vi "Snoothing.vi"(0 "Output 2":refnum<vi>, 2 "Value":i32, 3 "Delay (ms)":u32) -> (1 "Output":i32)   [LabVIEW 2015]
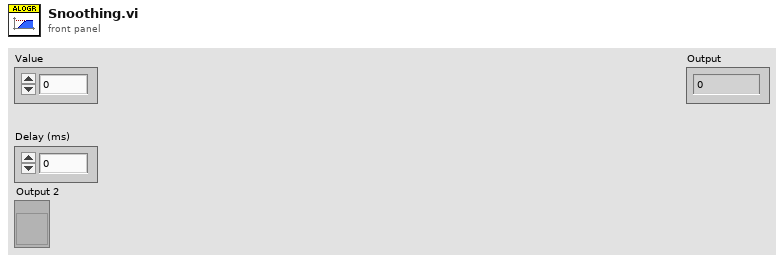
[diagram p1: front panel]
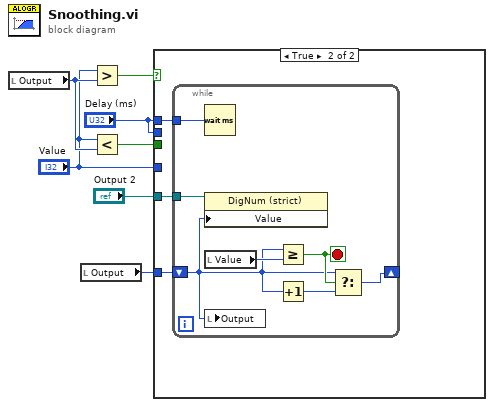
[diagram p0: block diagram]
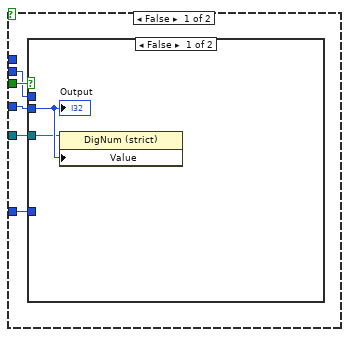
[diagram p2: hidden frame]
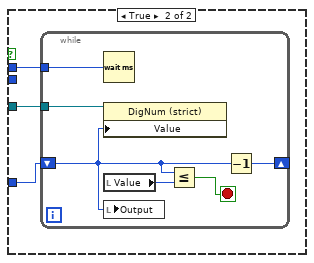
[diagram p3: hidden frame]
diagram:
  n1 = local read "Output"() -> (w6:i32)
  n2 = local read "Output"() -> (w4:i32)
  n3 = Greater?(x="Value", y=w6) -> (0:w7:bool)
  n4 = Less?(x="Value", y=w6) -> (x < y?=w5:bool)
  n5 = case shown="True" w7 {
    tunnel: w5 -> [w12 _]
    tunnel: w4 -> [w11 w26]
    tunnel: "Value" -> [w10 _]
    tunnel: "Delay (ms)" -> [w9 _]
    tunnel: "Delay (ms)" -> [_ w25]
    tunnel: "Output 2" -> [w8 w24]
    frame False {
      n6 = case shown="False" w12 {
        tunnel: w11 -> [_ w17]
        tunnel: w10 -> [w14 _]
        tunnel: w9 -> [_ w16]
        tunnel: w8 -> [w13 w15]
        frame False {
          n7 = property class="DigNum (strict)"(reference=w13, "Value"=w14) -> ()  [unwired: 1 in, 2 out]
          "Output" <- w14
        }
        frame True {
          n8 = while {
            shift-right: [w23] -> _
            shift-left: w17 -> [w19]
            tunnel: w16 -> [w20]
            tunnel: w15 -> [w18]
            stop <- w21 stop-if-true
            n9 = Wait (ms)(milliseconds to wait=w20) -> ()  [unwired: 1 out]
            n10 = property class="DigNum (strict)"(reference=w18, "Value"=w19) -> ()  [unwired: 1 in, 2 out]
            n11 = local read "Value"() -> (w22:i32)
            n12 = local write "Output"(w19) -> ()
            n13 = Less Or Equal?(x=w19, y=w22) -> (x <= y?=w21:bool)
            n14 = Decrement(x=w19) -> (x-1=w23:i32)
          }
        }
      }
    }
    frame True {
      n15 = while {
        shift-right: [w31] -> _
        shift-left: w26 -> [w27]
        tunnel: w25 -> [w29]
        tunnel: w24 -> [w28]
        stop <- w33 stop-if-true
        n16 = Wait (ms)(milliseconds to wait=w29) -> ()  [unwired: 1 out]
        n17 = property class="DigNum (strict)"(reference=w28, "Value"=w27) -> ()  [unwired: 1 in, 2 out]
        n18 = local read "Value"() -> (w30:i32)
        n19 = local write "Output"(w27) -> ()
        n20 = Greater Or Equal?(x=w27, y=w30) -> (x >= y?=w33:bool)
        n21 = Increment(x=w27) -> (x+1=w32:i32)
        n22 = Select(t=w27, s=w33, f=w32) -> (s? t:f=w31:i32)
      }
    }
  }
